vi "Cockpit UDP Send.vi"(8 "error in":errorcluster, 10 "write UDP array":sgl[](array[numeric]), 11 "connection ID":refnum<k16>) -> (0 "error out":errorcluster, 3 "connection ID out":refnum<k16>)   [LabVIEW 2010]
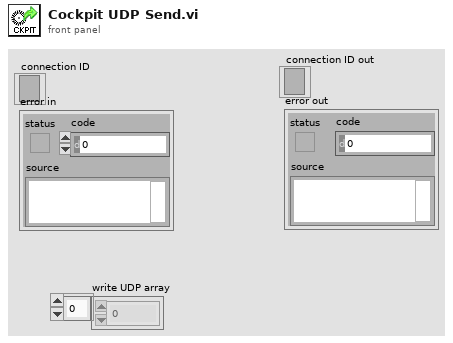
[diagram p1: front panel]
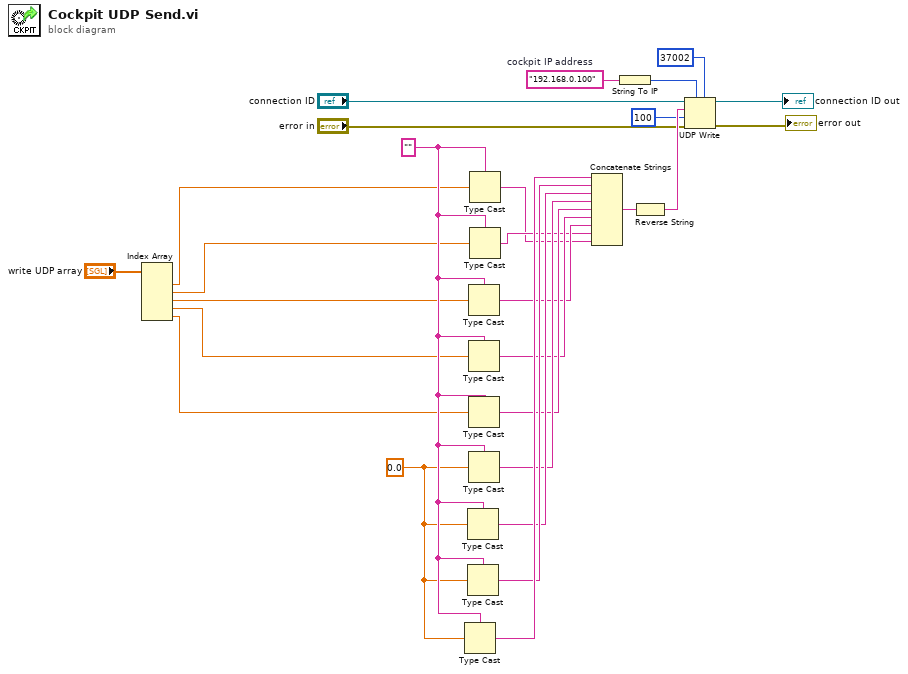
[diagram p0: block diagram]
diagram:
  w9 = sgl 0.0 ("enc 5")
  w12 = "192.168.0.100"  # cockpit IP address
  w23 = "" ("reversed")
  n1 = Index Array(array="write UDP array") -> (element #1=w8:sgl, element #2=w7:sgl, element #3=w6:sgl, element #4=w5:sgl, element #5=w4:sgl)  [unwired: 5 in]
  n2 = Type Cast(type=w23, x=w9) -> (*(type *) &x=w22:string)
  n3 = Type Cast(type=w23, x=w9) -> (*(type *) &x=w20:string)
  n4 = Type Cast(type=w23, x=w9) -> (*(type *) &x=w21:string)
  n5 = Type Cast(type=w23, x=w6) -> (*(type *) &x=w16:string)
  n6 = Type Cast(type=w23, x=w5) -> (*(type *) &x=w17:string)
  n7 = Type Cast(type=w23, x=w4) -> (*(type *) &x=w18:string)
  n8 = Type Cast(type=w23, x=w9) -> (*(type *) &x=w19:string)
  n9 = Type Cast(type=w23, x=w8) -> (*(type *) &x=w14:string)
  n10 = Type Cast(type=w23, x=w7) -> (*(type *) &x=w15:string)
  n11 = Concatenate Strings(w22, w21, w20, w19, w18, w17, w16, w15, w14) -> (w25:string)
  n12 = String To IP(1:w12) -> (0:w11:u32)
  n13 = Reverse String(1:w25) -> (0:w24:string)
  n14 = UDP Write(address=w11, port or service name=u16 37002, connection ID="connection ID", data in=w24, 8:"error in", 9:100 ("timeout ms (25000)")) -> (error out=→"error out":errorcluster, 3:→"connection ID out":refnum<k16>)
